vi "Project.vi"(8 "error in (no error)":errorcluster, 10 "type":i32(ring)=1448153088 items=["Volume"=1448153088, "Reconstruction"=1448153089]) -> (0 "error out":errorcluster, 3 "VGS_Project out":refnum<class "VGS_Project.lvclass">)   [LabVIEW 2022 SP3, in "LV_VGS.lvlib" / "VGS_Project.lvclass"]
uses:
  VGS_Project.lvclass
  VGS_Project.lvclass/VGS_Project.ctl
  C:/Users/Andrey/Documents/GitHub/LV_VGS/vgs_project.dll
  vgs_project.dll
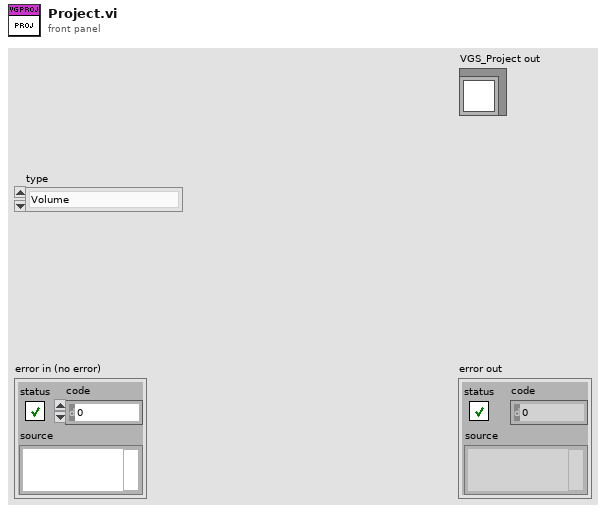
[diagram p1: front panel]
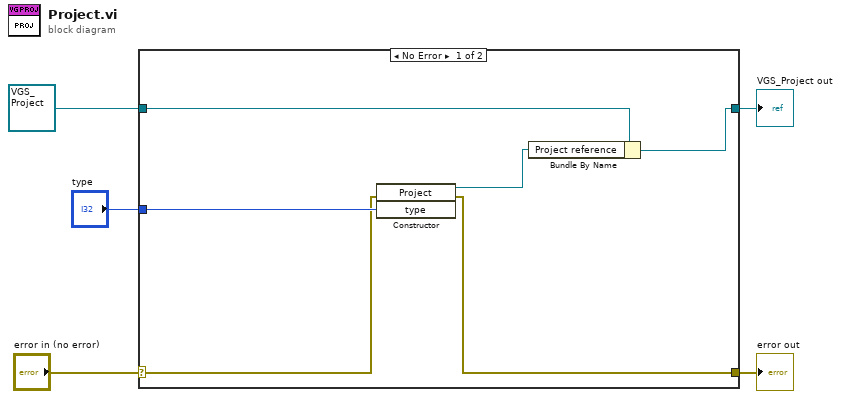
[diagram p0: block diagram]
diagram:
  n1 = case shown="No Error" "error in (no error)" {
    selector: "error in (no error)" -> [w7 w13]
    tunnel: [w6 w13] -> w4
    tunnel: [w8 w12] -> w2
    tunnel: refnum<class "VGS_Project.lvclass"> refnum ("VGS_Project in") -> [w10 w12]
    tunnel: "type" -> [w11 _]
    frame No Error {
      n2 = constructor class="Project"(error in=w7, "type"=w11) -> (reference out=w9:refnum<k24>, error out=w6:errorcluster)  [unwired: 2 in, 2 out]
      n3 = Bundle By Name(cluster=w10, "Project reference"=w9) -> (w8:refnum<class "VGS_Project.lvclass">)
    }
    frame Error {
    }
  }
  "error out" <- w4
  "VGS_Project out" <- w2
